vi "Create_Raw_data_file.vi"(0 "Setup filename":string, 1 "Start time":dbl, 2 "End time":dbl, 3 "No of averages":i32=1) -> (5 "Column headers":string[](array[string]), 7 "Values":string[][](array[string]), 8 "Error String":string)   [LabVIEW 2022 SP3]
uses:
  Controls/Post_Process.ctl
  Globals/Preference_global.vi
  Globals/Meas_global.vi
  Analysis/7 Hole Probe pressures to UVW/7HP_Global.vi
  Globals/Trav_pos_global.vi
  Globals/Constants_global.vi
panel:
  out "transposed array":string[][](array[string])
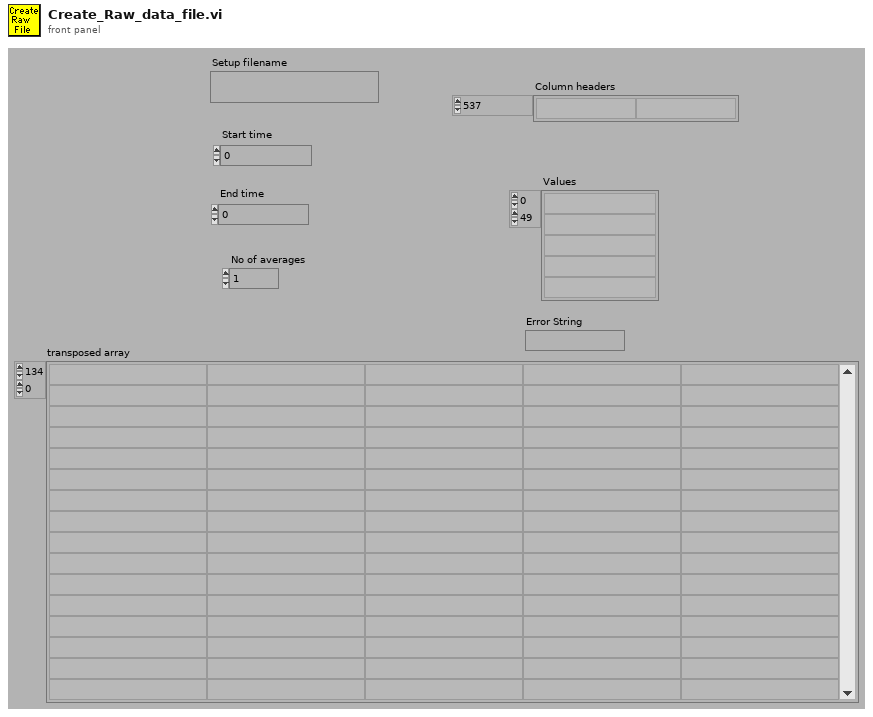
[diagram p1: front panel]
types:
  T1 = typedef "Post_Process.ctl" = enum16{"Take New Data", "Post Process Raw Data File"}
  T2 = typedef "Server_Comms.ctl" = enum16{"Do Not Link To Server", "Server Link Healthy"}
  T3 = typedef "Analysis_info_cluster.ctl" = cluster{"Colour":u32, "Inst type":T4, "Inst name":string, "Symbol":string, "Code name":string, "Extra Info":string, "Inst Array":T5, "U":dbl, "u^2":dbl, "u^3":dbl, "u^4":dbl, "Skew_u":dbl, "Kurt_u":dbl, "Sd Error in Mean":dbl, "% u'/U":dbl, "X":dbl, "Y":dbl, "Z":dbl, "Timescale integral Estimate":dbl, "Sd Error in Variance":dbl, "Calib File":path, "Calib Constants":dbl[], "Output Position":bool, "Stats":enum16{"None", "Basic", "Full"}, "Av Sampling Rate":dbl, "Av No of Samples":dbl, "Total Meas Time (s)":dbl, "OrigChName":string, "Max value":dbl, "Min value":dbl, "Req Sample Rate Hz":dbl, "Sync Delay Time (s)":dbl, "Ch No":i16, "Device":string, "Use Latest Calib":bool, "Port":string, "Metadata Ch Names":string[], "Metadata Ch Values":string[], "Label":string, "chState":T6, "Point Drift":dbl, "inputConfig":string}
  T4 = typedef "Inst_type.ctl" = enum16{"Raw voltage", "Raw with zero offsetting", "Propeller anemometer", "Pressure Transducer", "Pitot-static tube", "Hot wire", "Cross wire 1", "Cross wire 2", "Generic Linear", "Generic Polynomial", "Generic BackPoly", "Fast FID", "Thermocouple", "Cold wire", "Pulsed Wire", "LDA Vel", "LDA Tran time", "LDA Arr time", "Microphone"}
  T5 = typedef "Instrument_Array.ctl" = enum16{"PWA", "LDA", "Analogue"}
  T6 = typedef "channelState.ctl" = enum32{"No Selection", "Solo", "Mute"}
  T7 = typedef "Device ID port info.ctl" = cluster{"Ch No":i16[], "Req Sampling Rate":dbl[], "Port":string, "Index":i32[]}
  T8 = cluster{"Pressure Ch Names":string[], "Pressure Index":i32[], "Metadata Index":i32[], "Port":string}[]
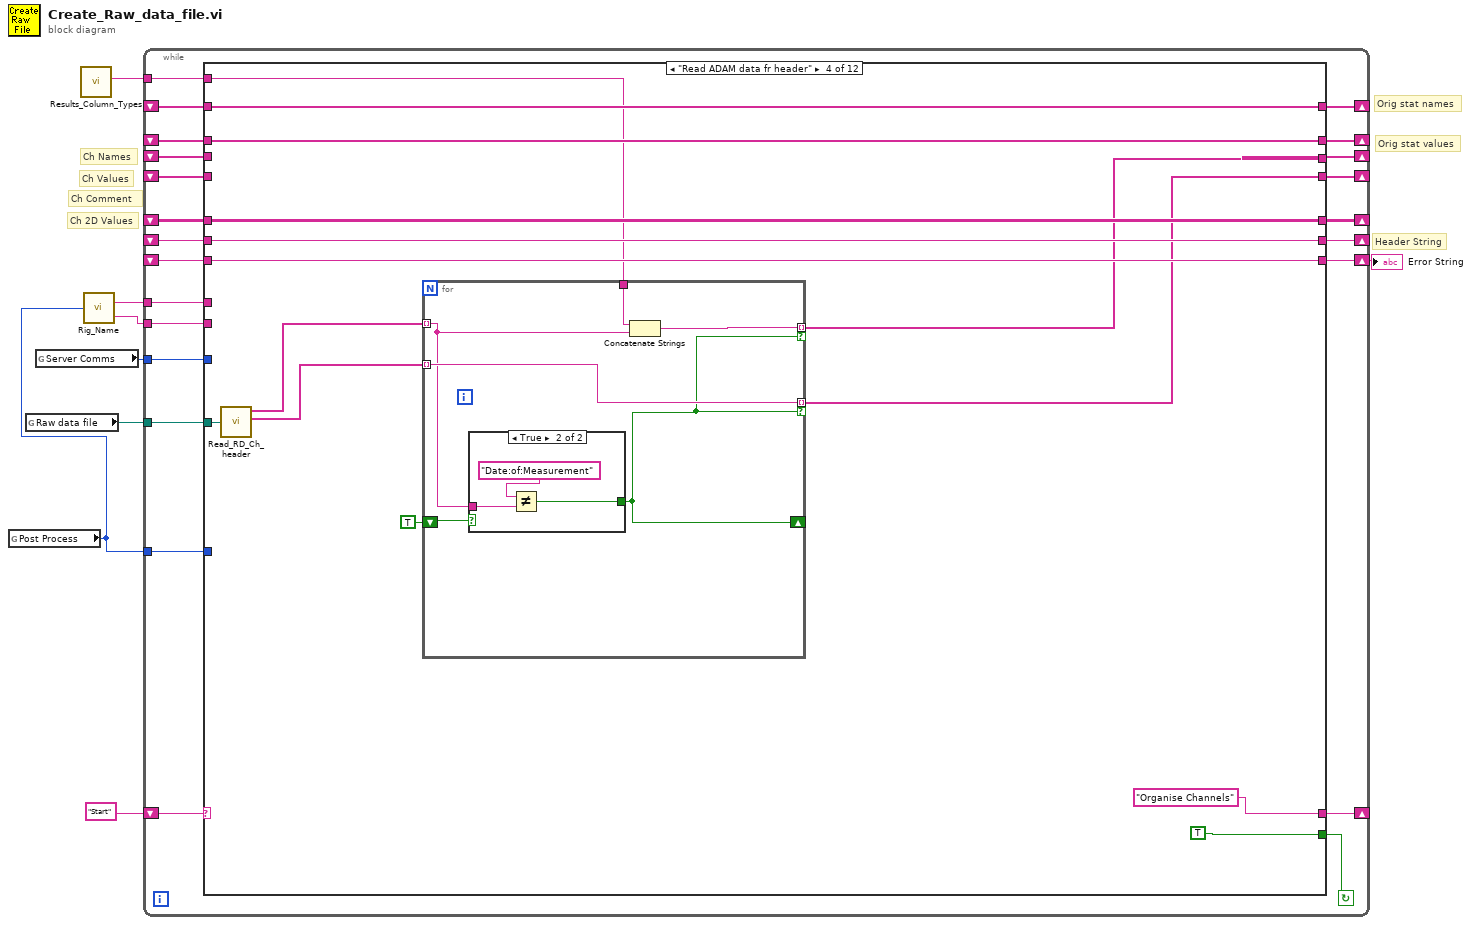
[diagram p0: block diagram]
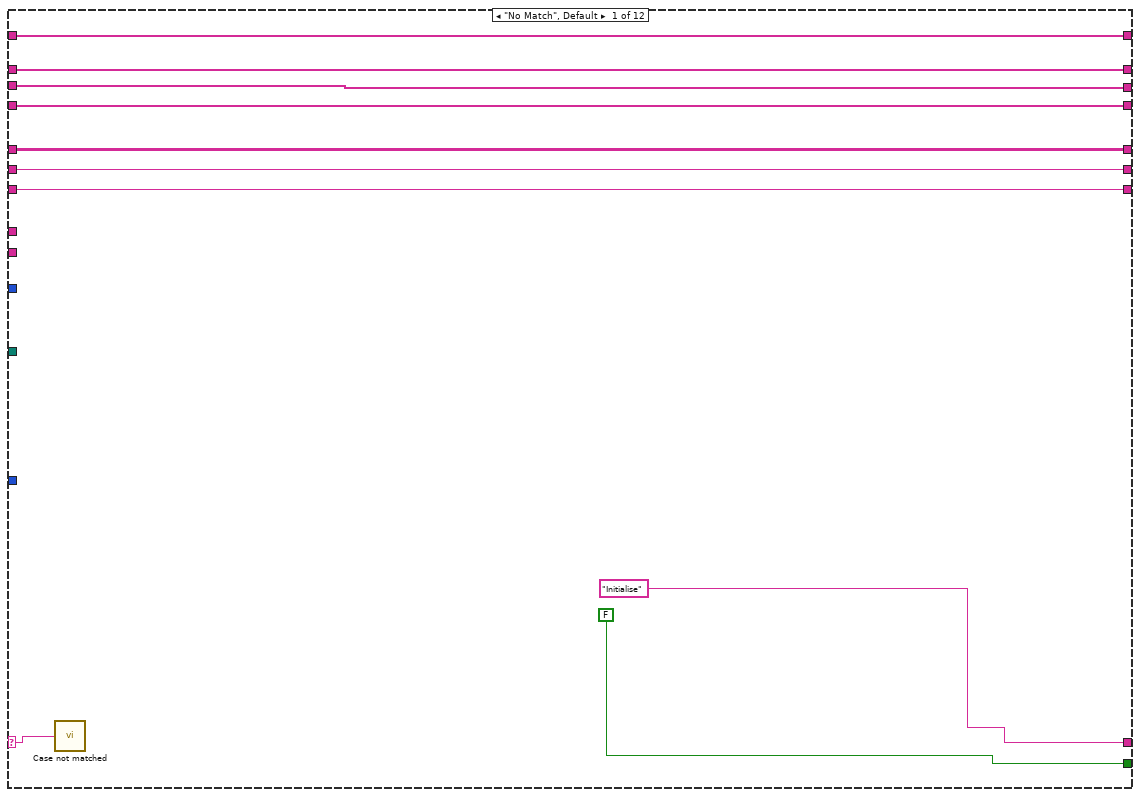
[diagram p2: hidden frame]
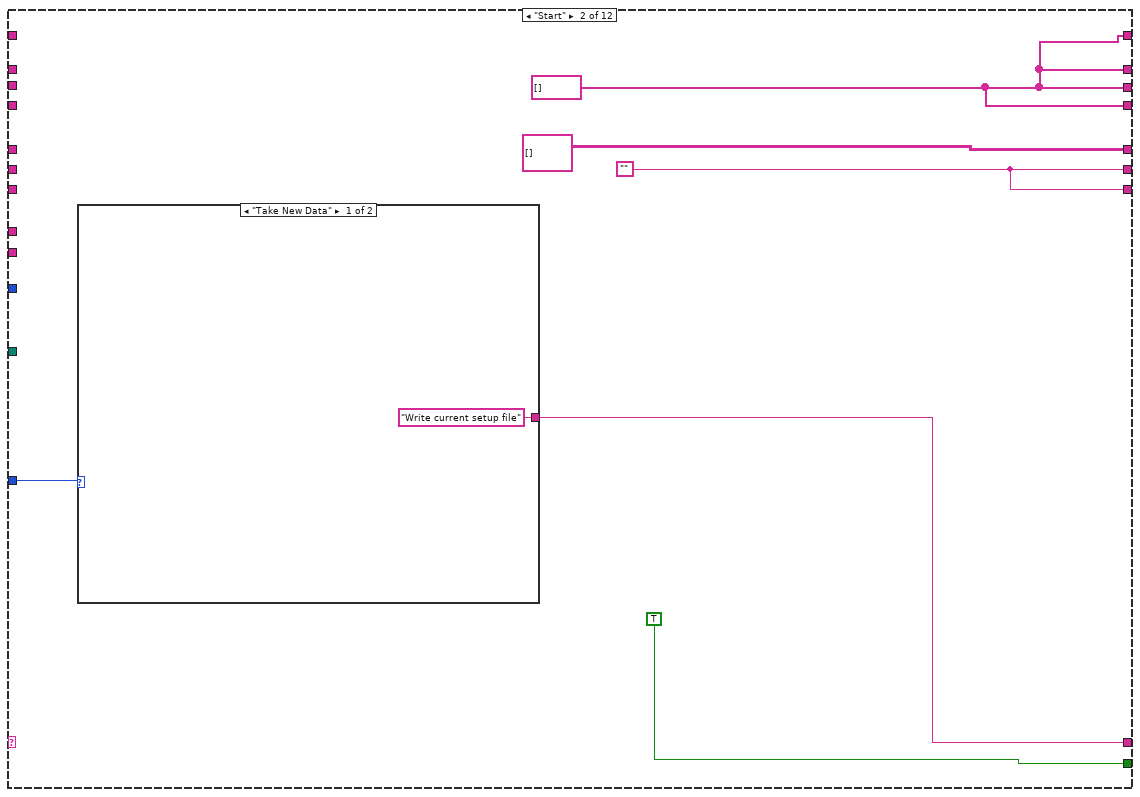
[diagram p3: hidden frame]
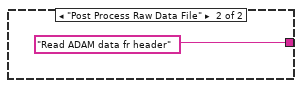
[diagram p4: hidden frame]
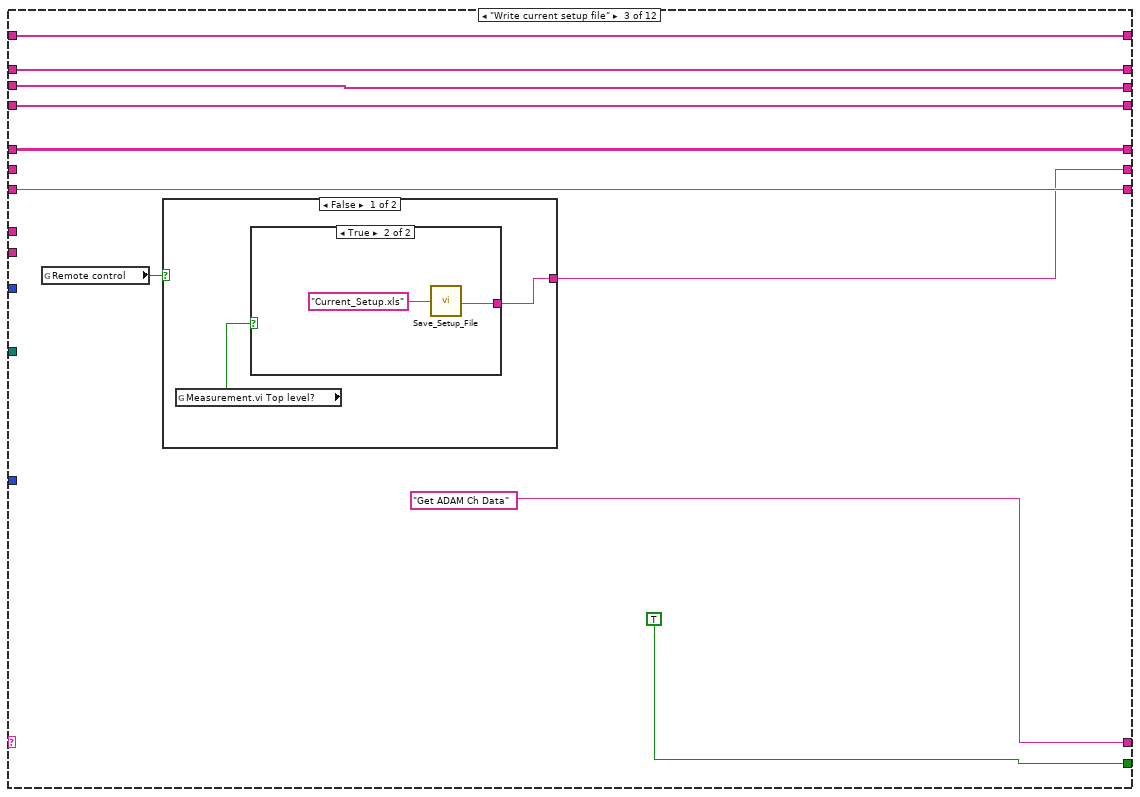
[diagram p5: hidden frame]
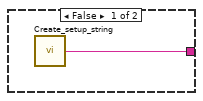
[diagram p6: hidden frame]
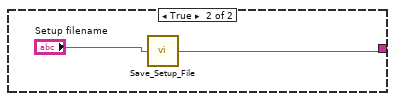
[diagram p7: hidden frame]
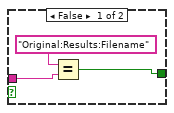
[diagram p8: hidden frame]
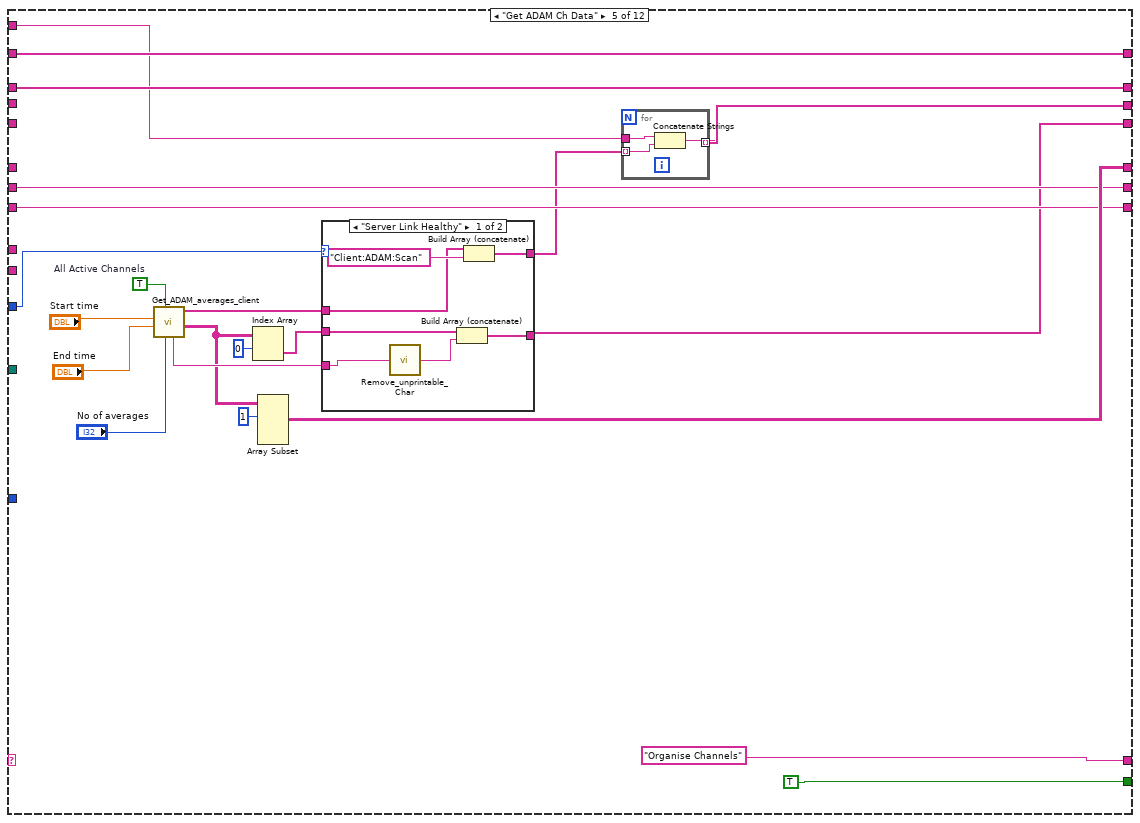
[diagram p9: hidden frame]
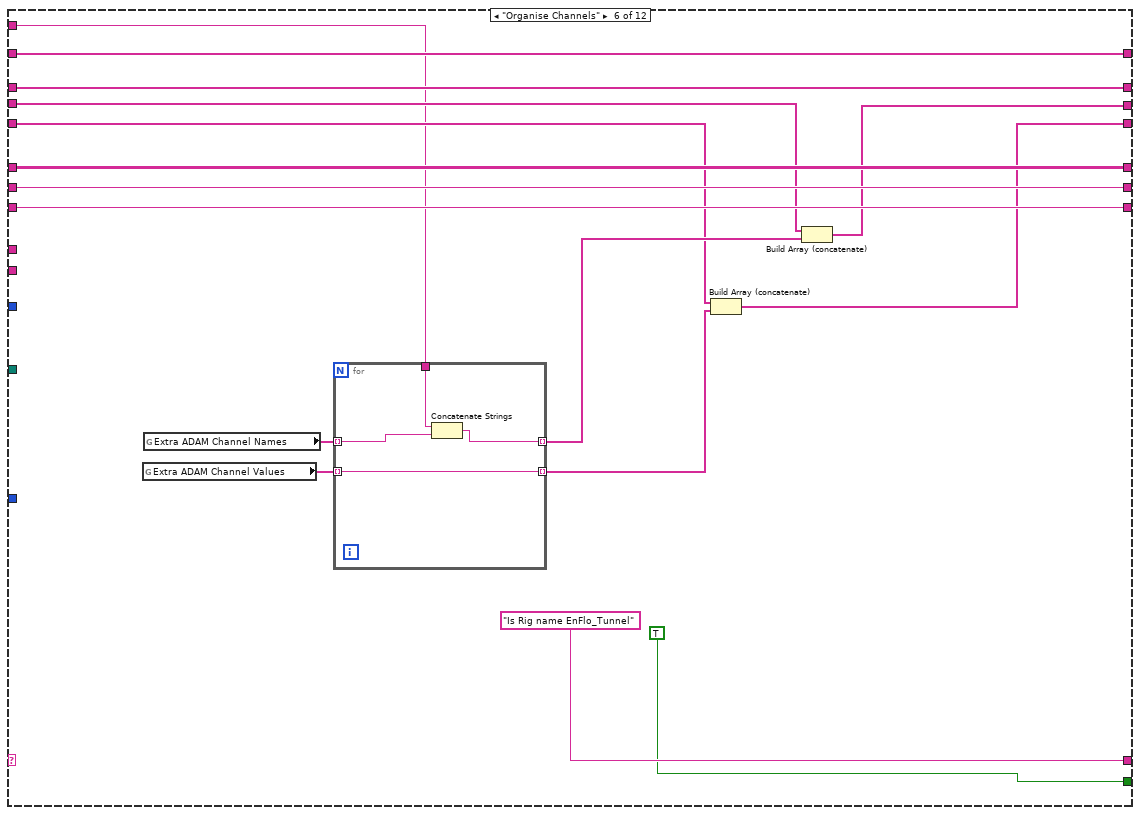
[diagram p11: hidden frame]
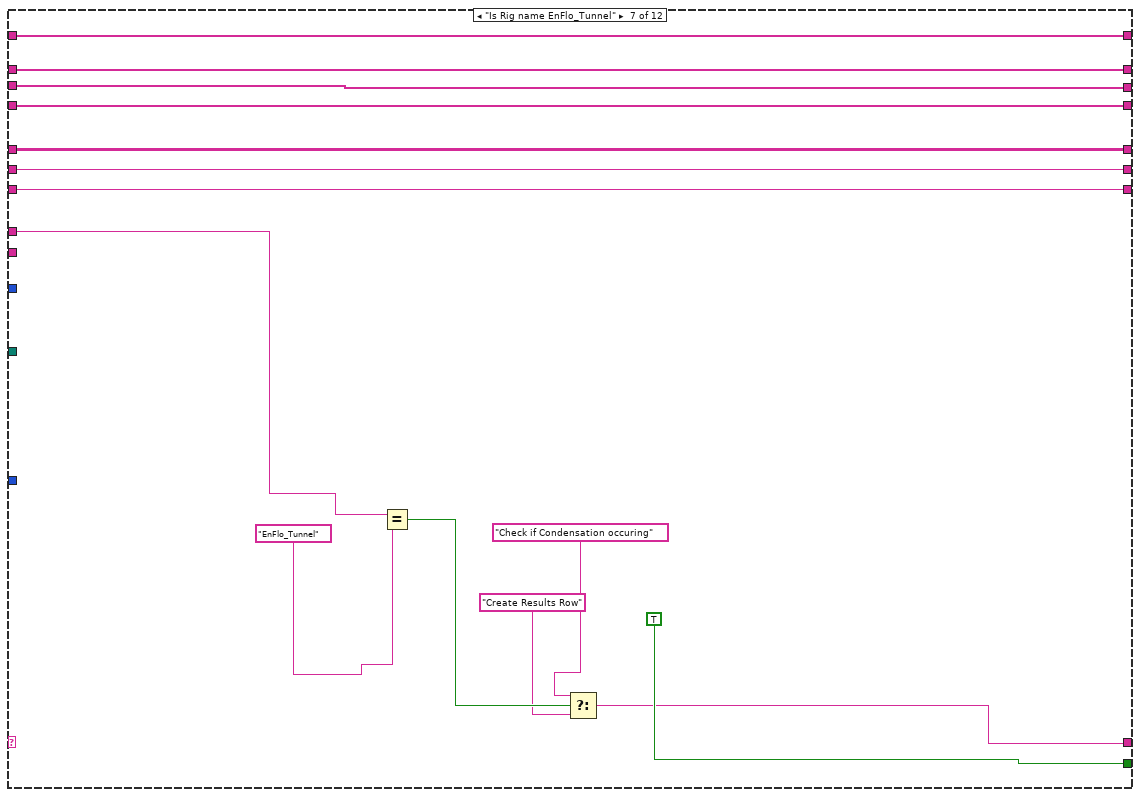
[diagram p12: hidden frame]
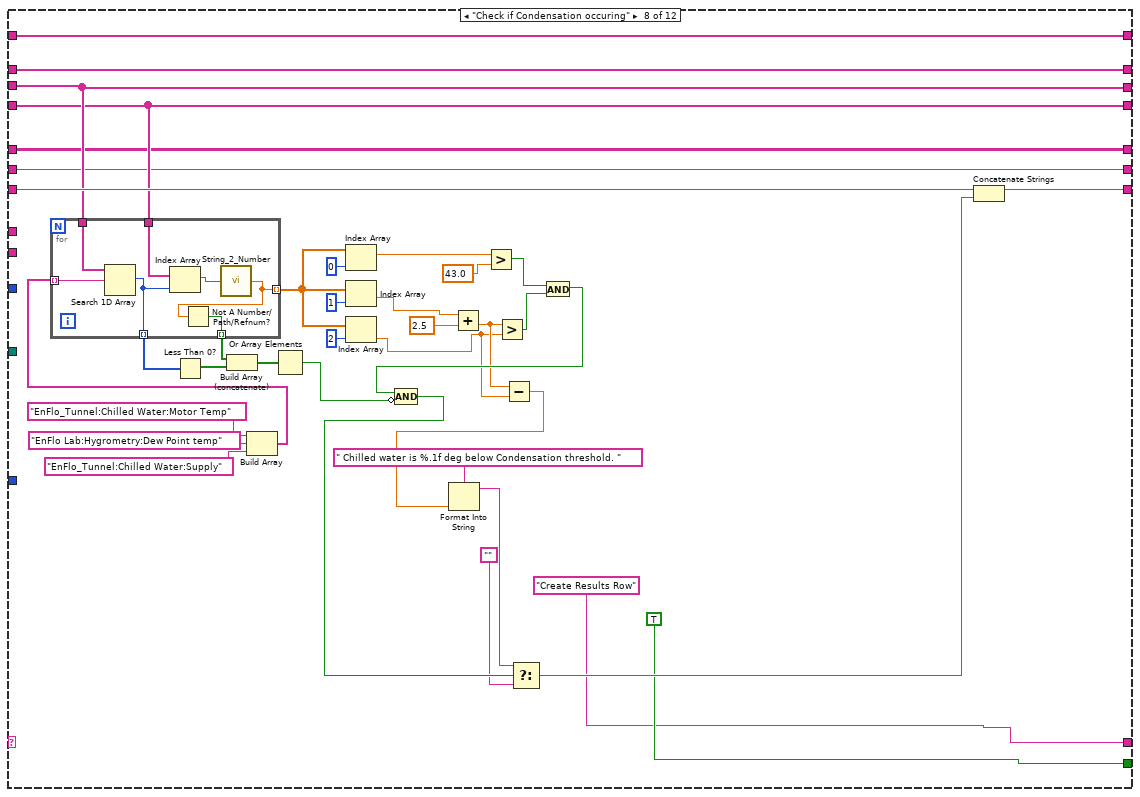
[diagram p13: hidden frame]
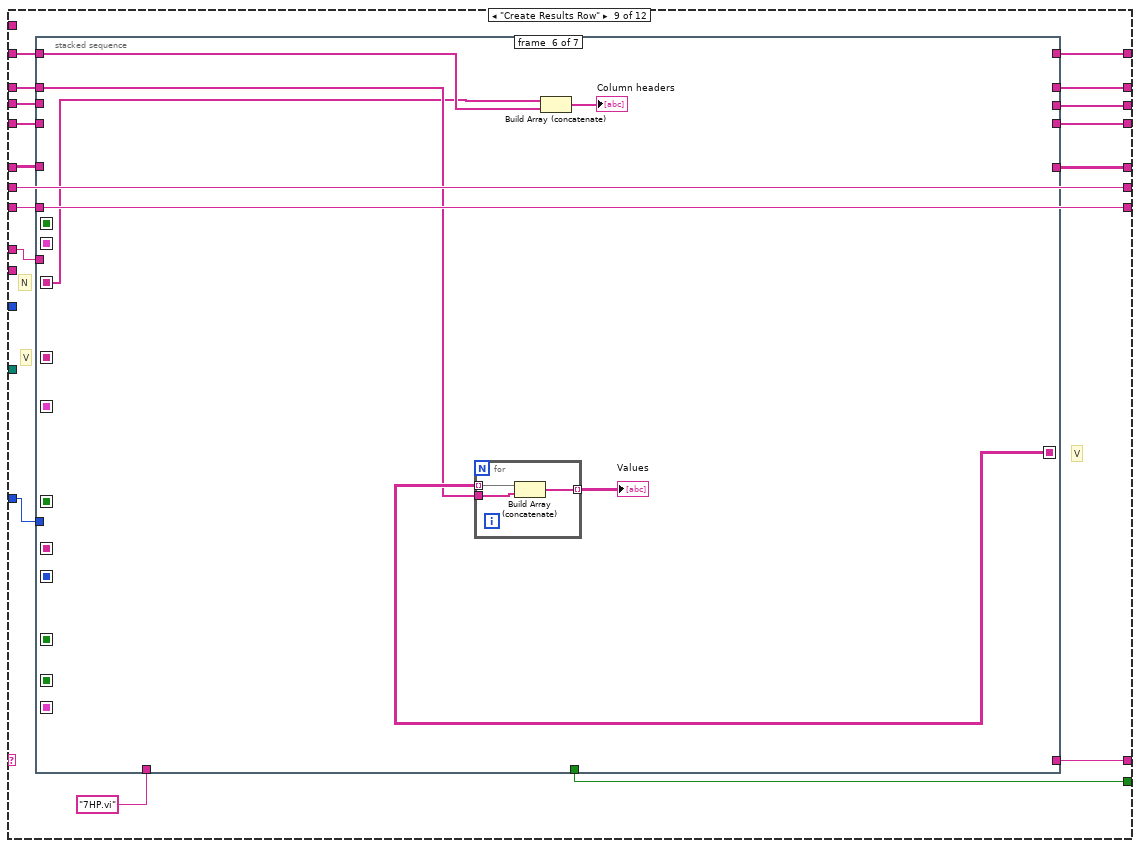
[diagram p14: hidden frame]
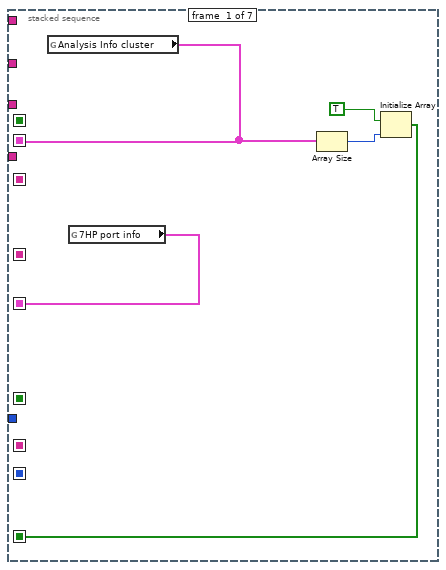
[diagram p15: hidden frame]
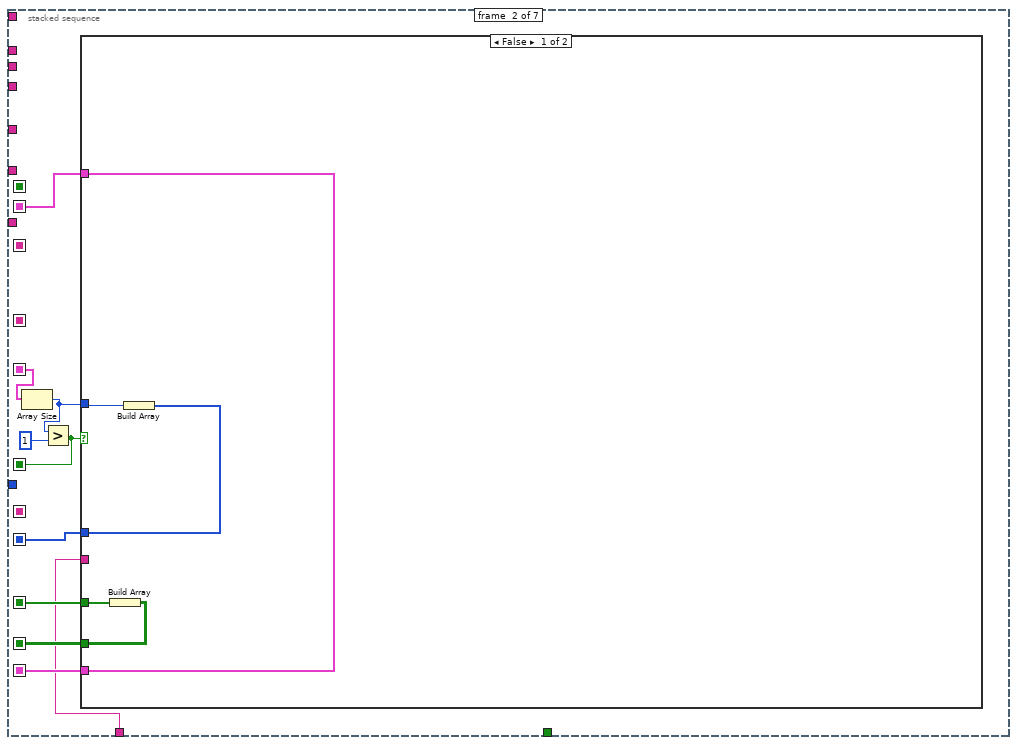
[diagram p16: hidden frame]
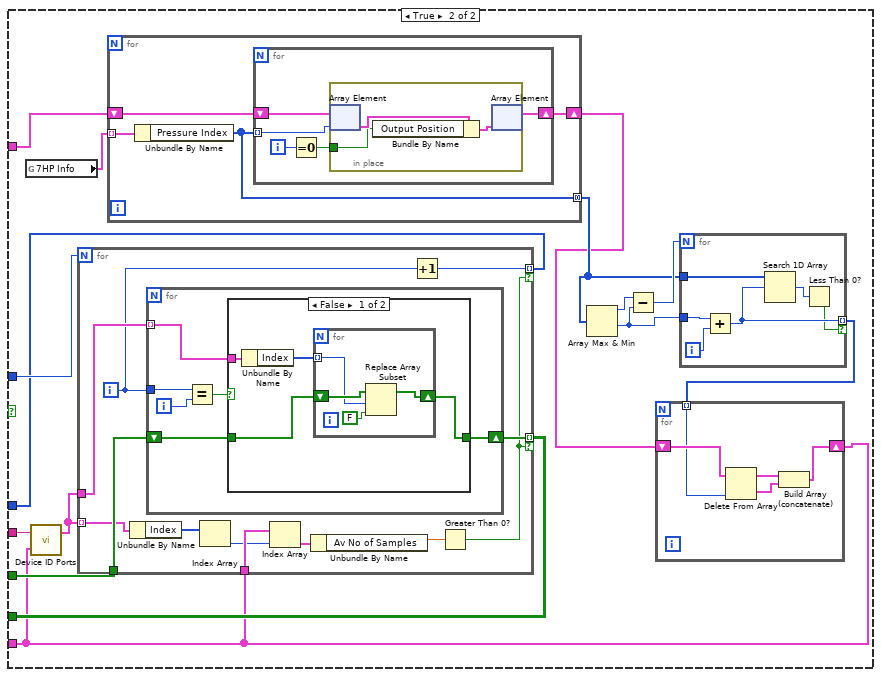
[diagram p17: hidden frame]
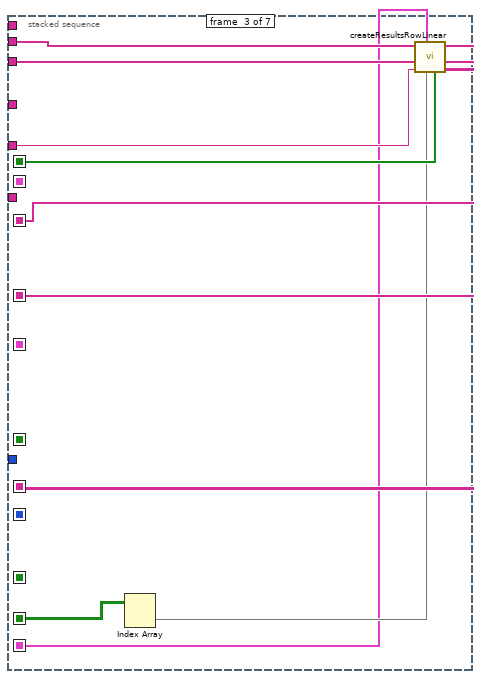
[diagram p19: hidden frame]
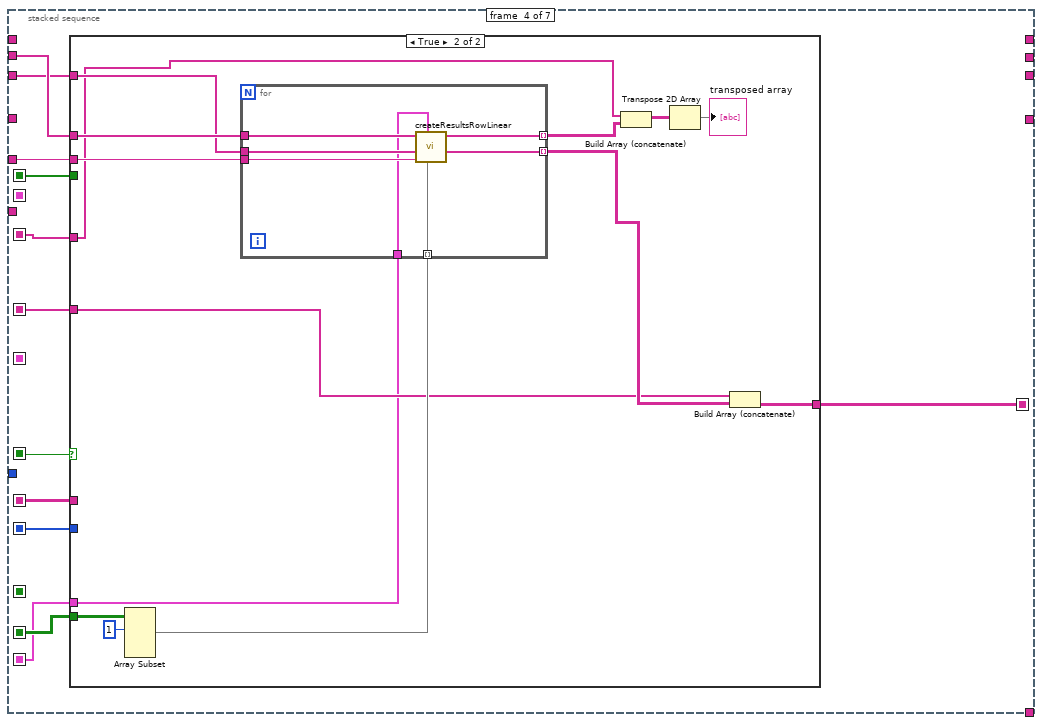
[diagram p20: hidden frame]
diagram:
  # "Orig stat values"
  # "Orig stat names"
  # "Header String"
  # "Ch 2D Values"
  # "Ch Comment"
  # "Ch Values"
  # "Ch Names"
  n1 = global read "Meas_global.vi" "Post Process"() -> (w4:T1)
  n2 = global read "Meas_global.vi" "Raw data file"() -> (w7:path)
  n3 = global read "Preference_global.vi" "Server Comms"() -> (w6:T2)
  n4 = call "Results_Column_Types.vi"() -> ("Metadata"=w1:string)  [unwired: 9 in, 2 out]
  n5 = call "Rig_Name.vi"("Post Process"=w4) -> ("Rig Setup before dash"=w3:string, "Hard Disk name"=w2:string)
  n6 = while {
    tunnel: w6 -> [w16]
    tunnel: w7 -> [w17]
    tunnel: w4 -> [w18]
    shift-left: _ -> [w20]
    shift-right: [w19] -> _
    shift-left: _ -> [w25]
    shift-right: [w24] -> w5
    shift-left: _ -> [w21]
    shift-right: [w26] -> _
    shift-left: _ -> [w22]
    shift-right: [w27] -> _
    shift-left: _ -> [w23]
    shift-right: [w28] -> _
    shift-left: "Start" -> [w29]
    shift-right: [w30] -> _
    tunnel: w3 -> [w15]
    tunnel: w2 -> [w14]
    shift-right: [w10] -> _
    shift-left: _ -> [w11]
    shift-right: [w12] -> _
    shift-left: _ -> [w13]
    tunnel: w1 -> [w9]
    stop <- w31 continue-if-true
    n7 = case shown="\"Read ADAM data fr header\"" w29 {
      selector: w29 -> [w32 _ _ _ _ _ _ _ _ _ _ _]
      tunnel: [FALSE TRUE TRUE TRUE TRUE TRUE TRUE TRUE w212 TRUE TRUE FALSE] -> w31
      tunnel: ["Initialise" w43 "Get ADAM Ch Data" "Organise Channels" "Organise Channels" "Is Rig name EnFlo_Tunnel" w153 "Create Results Row" w222 "Add Raw Data header info" "Add Raw Data fr Tempory file" "End"] -> w30
      tunnel: [w39 w42 w59 w73 w94 w134 w160 w168 w219 w436 w471 w487] -> w28
      tunnel: [w38 w42 w58 w72 w96 w128 w159 w167 w214 w451 w472 w488] -> w27
      tunnel: [w37 string[][] [] w57 w78 w102 w140 w158 w166 w216 w444 w473 w489] -> w26
      tunnel: w25 -> [w36 _ w55 w79 w101 w138 w155 w171 w220 w455 w474 w490]
      tunnel: [w36 w45 w55 w79 w101 w138 w155 w169 w220 w455 w474 w490] -> w24
      tunnel: w23 -> [w39 _ w59 _ _ w135 w160 w168 w218 w436 w471 w487]
      tunnel: w22 -> [w38 _ w58 _ _ w129 w159 w167 w215 w451 w472 w488]
      tunnel: w21 -> [w37 _ w57 w78 _ w140 w158 w166 w217 w444 w473 w489]
      tunnel: w20 -> [w35 _ _ w77 w100 w139 w156 w164 w221 w437 w465 w481]
      tunnel: [w35 w45 w50 w77 w100 w139 w156 w164 w221 w448 w468 ""] -> w19
      tunnel: w18 -> [_ w44 _ _ _ _ _ _ w213 _ _ _]
      tunnel: w17 -> [_ _ _ w76 _ _ _ _ _ _ _ w478]
      tunnel: w16 -> [_ _ _ _ w99 _ _ _ _ _ _ _]
      tunnel: w15 -> [_ _ _ _ _ _ w150 _ w211 _ _ _]
      tunnel: w14 -> [_ _ _ _ _ _ _ _ _ _ _ _]
      tunnel: w13 -> [w34 _ w52 w69 w98 w137 w148 w163 w209 w439 w467 w483]
      tunnel: [w34 w42 w52 w69 w98 w137 w148 w163 w210 w439 w467 w483] -> w12
      tunnel: w11 -> [w33 _ w51 w70 w97 w136 w147 w162 w207 w438 w466 w482]
      tunnel: [w33 w42 w51 w70 w97 w136 w147 w162 w208 w438 w466 w482] -> w10
      tunnel: w9 -> [_ _ _ w67 w93 w127 _ _ _ _ _ _]
      frame "No Match", Default {
        n8 = call "Case not matched.vi"("Case Name not Matched"=w32) -> ()
      }
      frame "Start" {
        w45 = ""
        w42 = string[] []
        n9 = case shown="\"Take New Data\"" w44 {
          tunnel: ["Write current setup file" "Read ADAM data fr header"] -> w43
          frame "Take New Data" {
          }
          frame "Post Process Raw Data File" {
          }
        }
      }
      frame "Write current setup file" {
        n10 = global read "Meas_global.vi" "Remote control"() -> (w54:bool)
        n11 = case shown="False" w54 {
          tunnel: [w61 w65] -> w50
          frame False {
            n12 = global read "Meas_global.vi" "Measurement.vi Top level?"() -> (w60:bool)
            n13 = case shown="True" w60 {
              tunnel: [w62 w64] -> w61
              frame False {
                n14 = call "Create_setup_string.vi"() -> ("Setup String"=w62:string)  [unwired: 1 out]
              }
              frame True {
                n15 = call "Save_Setup_File.vi"("Setup filename"="Current_Setup.xls") -> ("Setup String"=w64:string)
              }
            }
          }
          frame True {
            n16 = call "Save_Setup_File.vi"("Setup filename"="Setup filename") -> ("Setup String"=w65:string)
          }
        }
      }
      frame "Read ADAM data fr header" {
        n17 = call "Read_RD_Ch_header.vi"("Raw data file"=w76) -> ("Ch Name Out"=w75:string[], "Ch Values"=w74:string[])  [unwired: 2 out]
        n18 = for {
          shift-right: [w84] -> _
          shift-left: TRUE -> [w86]
          tunnel: w75 -> [w83] mode=indexing
          tunnel: w74 -> [w85] mode=indexing
          tunnel: [w81] -> w73 mode=indexing if=w84
          tunnel: [w85] -> w72 mode=indexing if=w84
          tunnel: w67 -> [w82]
          n19 = case shown="True" w86 {
            tunnel: w83 -> [w88 w92]
            tunnel: [w87 w90] -> w84
            frame False {
              n20 = Equal?(x="Original:Results:Filename", y=w88) -> (x = y?=w87:bool)
            }
            frame True {
              n21 = Not Equal?(x="Date:of:Measurement", y=w92) -> (x != y?=w90:bool)
            }
          }
          n22 = Concatenate Strings(w82, w83) -> (w81:string)
        }
      }
      frame "Get ADAM Ch Data" {
        w106 = TRUE  # All Active Channels
        n23 = call "Get_ADAM_averages_client.vi"("No of averages"="No of averages", "All Active Channels"=w106, "End time"="End time", "Start time"="Start time") -> ("Values"=w109:string[][], "Titles"=w111:string[], "Messages"=w112:string)  [unwired: 1 in, 4 out]
        n24 = Index Array(array=w109, index (row)=0 ("Index")) -> (element=w103:string[])  [unwired: 1 in]
        n25 = Array Subset(array=w109, index (row)=1 ("Array Index")) -> (w102:string[][])  [unwired: 3 in]
        n26 = case shown="\"Server Link Healthy\"" w99 {
          tunnel: w112 -> [w119 _]
          tunnel: w111 -> [w123 w126]
          tunnel: [w122 w126] -> w95
          tunnel: [w121 w125] -> w96
          tunnel: w103 -> [w120 w125]
          frame "Server Link Healthy" {
            n27 = call "Remove_unprintable_Char.vi"("Input String"=w119) -> ("Output String"=w118:string)
            n28 = Build Array (concatenate)(w120, w118) -> (w121:string[])
            n29 = Build Array (concatenate)(w123, "Client:ADAM:Scan") -> (w122:string[])
          }
          frame "Do Not Link To Server" {
          }
        }
        n30 = for {
          tunnel: w95 -> [w117] mode=indexing
          tunnel: [w116] -> w94 mode=indexing
          tunnel: w93 -> [w115]
          n31 = Concatenate Strings(w115, w117) -> (w116:string)
        }
      }
      frame "Organise Channels" {
        n32 = global read "Meas_global.vi" "Extra ADAM Channel Values"() -> (w132:string[])
        n33 = global read "Meas_global.vi" "Extra ADAM Channel Names"() -> (w133:string[])
        n34 = for {
          tunnel: [w143] -> w131 mode=indexing
          tunnel: w133 -> [w145] mode=indexing
          tunnel: [w146] -> w130 mode=indexing
          tunnel: w132 -> [w146] mode=indexing
          tunnel: w127 -> [w144]
          n35 = Concatenate Strings(w144, w145) -> (w143:string)
        }
        n36 = Build Array (concatenate)(w129, w130) -> (w128:string[])
        n37 = Build Array (concatenate)(w135, w131) -> (w134:string[])
      }
      frame "Is Rig name EnFlo_Tunnel" {
        n38 = Equal?(x=w150, y="EnFlo_Tunnel") -> (x = y?=w154:bool)
        n39 = Select(t="Check if Condensation occuring", s=w154, f="Create Results Row") -> (s? t:f=w153:string)
      }
      frame "Check if Condensation occuring" {
        n40 = Build Array("EnFlo_Tunnel:Chilled Water:Motor Temp", "EnFlo Lab:Hygrometry:Dew Point temp", "EnFlo_Tunnel:Chilled Water:Supply") -> (w194:string[])
        n41 = for {
          tunnel: w168 -> [w205]
          tunnel: w194 -> [w204] mode=indexing
          tunnel: w167 -> [w203]
          tunnel: [w201] -> w195 mode=indexing
          tunnel: [w200] -> w193 mode=indexing
          tunnel: [w199] -> w186 mode=indexing
          n42 = Search 1D Array(1D array=w205, element=w204) -> (index of element=w201:i32)  [unwired: 1 out]
          n43 = Index Array(array=w203, index=w201) -> (element=w202:string)
          n44 = call "String_2_Number.vi"("Value"=w202) -> ("Numeric"=w200:dbl)
          n45 = Not A Number/Path/Refnum?(number/path/refnum=w200) -> (NaN/Path/Refnum?=w199:bool)
        }
        n46 = Less Than 0?(x=w195) -> (x < 0?=w185:bool[])
        n47 = Build Array (concatenate)(w186, w185) -> (w184:bool[])
        n48 = Or Array Elements(Boolean array=w184) -> (logical OR=w180:bool)
        n49 = Index Array(array=w193, index=0 ("Index")) -> (element=w187:dbl)
        n50 = Index Array(array=w193, index=1 ("Index")) -> (element=w183:dbl)
        n51 = Index Array(array=w193, index=2 ("Index")) -> (element=w175:dbl)
        n52 = Add(x=w183, y=2.5) -> (x+y=w176:dbl)
        n53 = Greater?(x=w187, y=43.0) -> (0:w181:bool)
        n54 = Greater?(x=w176, y=w175) -> (0:w182:bool)
        n55 = Subtract(x=w176, y=w175) -> (x-y=w174:dbl)
        n56 = Format Into String(format string=" Chilled water is %.1f deg below Condensation threshold. " ("Format String"), w174) -> (resulting string=w172:string)  [unwired: 2 in, 1 out]
        n57 = And(x=w181, y=w182) -> (x .and. y?=w179:bool)
        n58 = Compound Arithmetic op=AND(w179, invert w180) -> (w178:bool)
        n59 = Select(t=w172, s=w178, f="") -> (s? t:f=w170:string)
        n60 = Concatenate Strings(w171, w170) -> (w169:string)
      }
      frame "Create Results Row" {
        # "V"
        # "N"
        # "V"
        n61 = stacked-sequence {
          seq-local: [_ _ w315 _ _ _ _] -> [_ _ _ w320 w392 w417 _]
          seq-local: [_ _ w314 _ _ _ _] -> [_ _ _ w323 w389 _ _]
          seq-local: [_ _ w312 _ _ _ _] -> [_ _ _ w324 _ _ _]
          seq-local: [_ _ _ w321 _ _ _] -> [_ _ _ _ _ w420 _]
          seq-local: [_ _ w313 _ _ _ _] -> [_ _ _ w322 _ _ _]
          seq-local: [w227 _ _ _ _ _ _] -> [_ w236 _ _ _ _ _]
          seq-local: [w224 _ _ _ _ _ _] -> [_ w235 _ _ _ _ _]
          seq-local: [_ w234 _ _ _ _ _] -> [_ _ w310 w326 _ _ _]
          seq-local: [_ w233 _ _ _ _ _] -> [_ _ _ w325 _ _ _]
          seq-local: [w223 _ _ _ _ _ _] -> [_ w232 _ _ _ _ _]
          seq-local: [_ w231 _ _ _ _ _] -> [_ _ w308 w319 _ _ _]
          seq-local: [_ w228 _ _ _ _ _] -> [_ _ _ w318 _ _ _]
          tunnel: [_ _ _ _ _ _ "Add Adam Chs to header"] -> w222
          tunnel: w218 -> [_ _ w317 w329 w391 _ _]
          tunnel: w220 -> [_ _ w311 w327 _ _ _]
          tunnel: w215 -> [_ _ w316 w328 w388 _ _]
          tunnel: w217 -> [_ _ _ _ _ _ w431]
          tunnel: [_ _ _ _ w390 _ _] -> w219
          tunnel: [_ _ _ _ _ _ w431] -> w216
          tunnel: [_ _ _ _ w387 _ _] -> w214
          tunnel: w213 -> [_ _ _ _ w386 _ w427]
          tunnel: [_ _ _ _ _ _ w426] -> w212
          tunnel: w211 -> [_ _ _ _ _ _ _]
          tunnel: [_ _ _ _ _ _ w434] -> w210
          tunnel: w209 -> [_ _ _ _ _ w422 w434]
          tunnel: [_ _ _ _ _ _ w433] -> w208
          tunnel: w207 -> [_ _ _ _ _ w419 w433]
          tunnel: "7HP.vi" ("element") -> [_ w230 _ _ _ _ _]
          frame #0 {
            n62 = global read "Meas_global.vi" "Analysis Info cluster"() -> (w223:T3[])
            n63 = global read "7HP_Global.vi" "7HP port info"() -> (w227:T7[])
            n64 = Array Size(array=w223) -> (size(s)=w226:i32)
            n65 = Initialize Array(TRUE, w226) -> (w224:bool[])
          }
          frame #1 {
            n66 = Array Size(array=w236) -> (size(s)=w229:i32)
            n67 = Greater?(x=w229, y=1) -> (0:w233:bool)
            n68 = case shown="False" w233 {
              tunnel: w235 -> [w242 w257]
              tunnel: [w241 w256] -> w234
              tunnel: w232 -> [w240 w250]
              tunnel: [w240 w245] -> w231
              tunnel: w230 -> [_ w248]
              tunnel: w229 -> [w239 w246]
              tunnel: [w238 w243] -> w228
              frame False {
                n69 = Build Array(w242) -> (w241:bool[][])
                n70 = Build Array(w239) -> (w238:i32[])
              }
              frame True {
                n71 = global read "7HP_Global.vi" "7HP Info"() -> (w244:T8)
                n72 = for {
                  tunnel: w244 -> [w272] mode=indexing
                  shift-right: [w270] -> w249
                  shift-left: w250 -> [w271]
                  tunnel: [w269] -> w251 mode=concatenating
                  n73 = Unbundle By Name(w272) -> ("Pressure Index"=w269:i32[])
                  n74 = for {
                    shift-right: [w273] -> w270
                    shift-left: w271 -> [w277]
                    tunnel: w269 -> [w276] mode=indexing
                    i -> [w275]
                    n75 = Equal To 0?(x=w275) -> (x = 0?=w274:bool)
                    n76 = in-place {
                      in-place-border: w274 -> [w278]
                      n77 = in-place-array #1(w277, w276) -> (w280:T3)
                      n78 = Bundle By Name(cluster=w280, "Output Position"=w278) -> (w279:T3)
                      n79 = in-place-array #1(w279) -> (w273:T3[])  [unwired: 1 out]
                    }
                  }
                }
                n80 = Array Max & Min(array=w251) -> (max value=w255:i32, min value=w254:i32)  [unwired: 2 out]
                n81 = Subtract(x=w255, y=w254) -> (x-y=w253:i32)
                n82 = for {
                  N: w253 -> [_]
                  tunnel: w251 -> [w268]
                  tunnel: w254 -> [w266]
                  tunnel: [w265] -> w252 mode=indexing if=w263
                  i -> [w267]
                  n83 = Add(x=w266, y=w267) -> (x+y=w265:i32)
                  n84 = Search 1D Array(1D array=w268, element=w265) -> (index of element=w264:i32)  [unwired: 1 in]
                  n85 = Less Than 0?(x=w264) -> (x < 0?=w263:bool)
                }
                n86 = for {
                  shift-right: [w258] -> w245
                  shift-left: w249 -> [w262]
                  tunnel: w252 -> [w261] mode=indexing
                  n87 = Delete From Array(array=w262, index=w261) -> (deleted portion=w259:T3, array with subset deleted=w260:T3[])  [unwired: 1 in]
                  n88 = Build Array (concatenate)(w260, w259) -> (w258:T3[])
                }
                n89 = call "Device ID Ports.vi"("Analysis Info cluster"=w245, "DAQdeviceType"=w248) -> ("Device port info"=w247:T7[])  [unwired: 1 out]
                n90 = for {
                  N: w246 -> [_]
                  tunnel: w257 -> [w292]
                  tunnel: [w291] -> w256 mode=indexing if=w281
                  tunnel: w247 -> [w290]
                  tunnel: w247 -> [w289] mode=indexing
                  tunnel: w245 -> [w287]
                  tunnel: [w282] -> w243 mode=indexing if=w281
                  i -> [w283]
                  n91 = Unbundle By Name(w289) -> ("Index"=w288:i32[])
                  n92 = for {
                    tunnel: w290 -> [w293] mode=indexing
                    tunnel: w283 -> [w297]
                    shift-right: [w294] -> w291
                    shift-left: w292 -> [w295]
                    i -> [w298]
                    n93 = Equal?(x=w297, y=w298) -> (x = y?=w296:bool)
                    n94 = case shown="False" w296 {
                      tunnel: w295 -> [w302 w307]
                      tunnel: [w301 w307] -> w294
                      tunnel: w293 -> [w300 _]
                      frame False {
                        n95 = Unbundle By Name(w300) -> ("Index"=w299:i32[])
                        n96 = for {
                          shift-right: [w305] -> w301
                          shift-left: w302 -> [w306]
                          tunnel: w299 -> [w304] mode=indexing
                          n97 = Replace Array Subset(array=w306, new element=FALSE, index=w304) -> (w305:bool[])
                        }
                      }
                      frame True {
                      }
                    }
                  }
                  n98 = Index Array(array=w288) -> (element=w286:i32)  [unwired: 1 in]
                  n99 = Index Array(array=w287, index=w286) -> (element=w285:T3)
                  n100 = Unbundle By Name(w285) -> ("Av No of Samples"=w284:dbl)
                  n101 = Increment(x=w283) -> (x+1=w282:i32)
                  n102 = Greater Than 0?(x=w284) -> (x > 0?=w281:bool)
                }
              }
            }
          }
          frame #2 {
            n103 = Index Array(array=w310) -> (element=w309:bool[])  [unwired: 2 in]
            n104 = call "createResultsRowLinear.vi"("Indices to Output"=w309, "Analysis Info cluster"=w308, "Error String"=w311, "MetadataValuesIn"=w316, "MetadataNamesIn"=w317) -> ("row splitting"=w312:string[][], "Ch Values Out"=w314:string[], "Ch Names Out"=w315:string[], "Values to Keep in Dup rows"=w313:bool[])  [unwired: 3 in]
          }
          frame #3 {
            n105 = case shown="True" w325 {
              tunnel: w329 -> [_ w378]
              tunnel: w328 -> [_ w377]
              tunnel: w327 -> [_ w376]
              tunnel: w326 -> [_ w375]
              tunnel: w324 -> [w333 _]
              tunnel: w323 -> [w332 w370]
              tunnel: w322 -> [w331 _]
              tunnel: [w330 w371] -> w321
              tunnel: w320 -> [_ w368]
              tunnel: w319 -> [_ w369]
              tunnel: w318 -> [_ _]
              frame False {
                n106 = Array Size(array=w333) -> (size(s)=w337:i32[])
                n107 = Index Array(array=w337, index=0) -> (element=w335:i32)
                n108 = Greater Than 0?(x=w335) -> (x > 0?=w334:bool)
                n109 = case shown="True" w334 {
                  tunnel: w333 -> [_ w347]
                  tunnel: [w339 w346] -> w330
                  tunnel: w331 -> [_ w342]
                  tunnel: w332 -> [w338 w340]
                  frame False {
                    n110 = Build Array(w338) -> (w339:string[][])
                  }
                  frame True {
                    n111 = Array Size(array=w340) -> (size(s)=w345:i32)
                    n112 = Search 1D Array(1D array=w340, element="Instrument_name_place_holder") -> (index of element=w348:i32)  [unwired: 1 out]
                    n113 = Initialize Array(TRUE, w345) -> (w343:bool[])
                    n114 = Build Array (concatenate)(w342, w343) -> (w341:bool[])
                    n115 = for {
                      tunnel: w340 -> [w356]
                      tunnel: w348 -> [w355]
                      tunnel: w347 -> [w354] mode=indexing
                      tunnel: [w351] -> w346 mode=indexing
                      tunnel: w341 -> [w350]
                      i -> [w353]
                      n116 = Replace Array Subset(array=w356, new element=w354, index=w355) -> (w352:string[])
                      n117 = case shown="1, Default" w353 {
                        tunnel: w352 -> [w357 w359]
                        tunnel: [w357 w358] -> w351
                        tunnel: w350 -> [_ w360]
                        frame 0 {
                        }
                        frame 1, Default {
                          n118 = for {
                            tunnel: w360 -> [w364] mode=indexing
                            tunnel: w359 -> [w363] mode=indexing
                            tunnel: [w362] -> w358 mode=indexing
                            n119 = Select(t=w363, s=w364, f="") -> (s? t:f=w362:string)
                          }
                        }
                      }
                    }
                  }
                }
              }
              frame True {
                n120 = Array Subset(array=w375, index (row)=1 ("index")) -> (w373:bool[][])  [unwired: 3 in]
                n121 = for {
                  tunnel: w378 -> [w385]
                  tunnel: w377 -> [w384]
                  tunnel: w376 -> [w383]
                  tunnel: w373 -> [w382] mode=indexing
                  tunnel: [w381] -> w372 mode=indexing
                  tunnel: w369 -> [w380]
                  tunnel: [w379] -> w367 mode=indexing
                  n122 = call "createResultsRowLinear.vi"("Indices to Output"=w382, "Analysis Info cluster"=w380, "Error String"=w383, "MetadataValuesIn"=w384, "MetadataNamesIn"=w385) -> ("Ch Values Out"=w381:string[], "Ch Names Out"=w379:string[])  [unwired: 3 in, 2 out]
                }
                n123 = Build Array (concatenate)(w368, w367) -> (w366:string[][])
                n124 = Transpose 2D Array(2D array=w366) -> (transposed array=→"transposed array":string[][])
                n125 = Build Array (concatenate)(w370, w372) -> (w371:string[][])
              }
            }
          }
          frame #4 {
            n126 = case shown="\"Take New Data\"" w386 {
              tunnel: w392 -> [w398 _]
              tunnel: w391 -> [w397 w416]
              tunnel: [w396 w416] -> w390
              tunnel: w389 -> [w395 _]
              tunnel: w388 -> [w394 w415]
              tunnel: [w393 w415] -> w387
              frame "Take New Data" {
                n127 = for {
                  tunnel: w397 -> [w406]
                  tunnel: w398 -> [w402] mode=indexing
                  shift-right: [w403] -> w396
                  shift-left: w397 -> [w404]
                  shift-right: [w400] -> w393
                  shift-left: w394 -> [w401]
                  tunnel: w395 -> [w399] mode=indexing
                  n128 = Search 1D Array(1D array=w406, element=w402) -> (index of element=w405:i32)  [unwired: 1 out]
                  n129 = case shown="-1" w405 {
                    tunnel: w404 -> [w408 w414]
                    tunnel: [w408 w412] -> w403
                    tunnel: w402 -> [_ w413]
                    tunnel: w401 -> [w407 w410]
                    tunnel: [w407 w409] -> w400
                    tunnel: w399 -> [_ w411]
                    frame 0, Default {
                    }
                    frame -1 {
                      n130 = Build Array (concatenate)(w410, w411) -> (w409:string[])
                      n131 = Build Array (concatenate)(w414, w413) -> (w412:string[])
                    }
                  }
                }
              }
              frame "Post Process Raw Data File" {
              }
            }
          }
          frame #5 {
            n132 = for {
              tunnel: w420 -> [w425] mode=indexing
              tunnel: w419 -> [w424]
              tunnel: [w423] -> w418 mode=indexing
              n133 = Build Array (concatenate)(w425, w424) -> (w423:string[])
            }
            "Values" <- w418
            n134 = Build Array (concatenate)(w417, w422) -> (→"Column headers":string[])
          }
          frame #6 {
            n135 = global read "Trav_pos_global.vi" "Dummy Measurement?"() -> (w429:bool)
            n136 = Equal?(x=Post_Process."Take New Data" ("Post Process"), y=w427) -> (x = y?=w430:bool)
            n137 = Compound Arithmetic op=AND(invert w429, w430) -> (w426:bool)
          }
        }
      }
      frame "Add Adam Chs to header" {
        w440 = FALSE  # Email On Error?
        n138 = for {
          tunnel: w436 -> [w460] mode=indexing
          tunnel: [w458] -> w435 mode=indexing
          n139 = Match Pattern(string=w460, regular expression=":") -> (after substring=w458:string)  [unwired: 1 in, 3 out]
        }
        n140 = call "Channel_name_checker.vi"("Email On Error?"=w440, "Channel names"=w435) -> ("Channel names Out"=w441:string[])  [unwired: 1 out]
        n141 = for {
          tunnel: w441 -> [w464] mode=indexing
          tunnel: [w463] -> w454 mode=indexing
          tunnel: [w462] -> w453 mode=indexing
          tunnel: [w461] -> w452 mode=indexing
          n142 = call "Split_Ch_name.vi"("Ch name"=w464) -> ("Top level"=w463:string, "Middle"=w462:string, "Low level"=w461:string)
        }
        n143 = Array To Spreadsheet String(array=w444, 3:"%s" ("format string")) -> (spreadsheet string=w442:string)  [unwired: 1 out]
        n144 = Build Array(w454, w453, w452, w451) -> (w449:string[][])
        n145 = Array To Spreadsheet String(array=w449, 3:"%s" ("format string")) -> (spreadsheet string=w443:string)  [unwired: 1 out]
        n146 = Concatenate Strings(w443, w442, "***************************************" ("Substring"), "\r\n", w437) -> (w448:string)
      }
      frame "Add Raw Data header info" {
        n147 = String Length(string=w465) -> (length=w470:i32)
        n148 = call "Raw_Data_File_Start_text.vi"("Header length"=w470) -> ("Start String"=w469:string)
        n149 = Concatenate Strings(w469, w465) -> (w468:string)
      }
      frame "Add Raw Data fr Tempory file" {
        n150 = global read "Constants_global.vi" "Data Folder Local"() -> (w485:path)
        n151 = Build Path(base path=w485, name or relative path="Tempory_Raw_Data_File.xls") -> (appended path=w480:path)
        n152 = call "Read Characters with check.vi"("file (use dialog)"=w480) -> ("Read String"=w479:string)  [unwired: 1 in, 1 out]
        n153 = Concatenate Strings(w481, w479) -> (w477:string)
        n154 = call "Write Characters with check.vi"("String to Write"=w477, "file (use dialog)"=w478) -> ()  [unwired: 2 in, 1 out]
      }
    }
  }
  "Error String" <- w5
